vi "PH_AWG-510.Unpack Output Settings.vi"(2 "Output Settings":T1={"Activate Channel"=FALSE, "VPP (V)"=0.0, "Clock (Hz)"=0.0, "File Name (Device)"="", "#1"=0, "#2"=0, "#3"=0, "#4"=0, "#5"=0, "#6"=0, "#7"=0, "#8"=0, "#9"=0, "#10"=0, "#11"=0, "#12"=0, "#13"=0, "#14"=0, "#15"=0, "#16"=0, "#17"=0, "#18"=0, "#19"=0, "#20"=0, "Offset (V)"=-1.0} {"#20" max=1023 step=1 scale=0.0..1023.0; "#19" max=1023 step=1 scale=0.0..1023.0; "#18" max=1023 step=1 scale=0.0..1023.0; "#17" max=1023 step=1 scale=0.0..1023.0; "#16" max=1023 step=1 scale=0.0..1023.0; "#15" max=1023 step=1 scale=0.0..1023.0; "#14" max=1023 step=1 scale=0.0..1023.0; "#13" max=1023 step=1 scale=0.0..1023.0; "#12" max=1023 step=1 scale=0.0..1023.0; "#11" max=1023 step=1 scale=0.0..1023.0; "#10" max=1023 step=1 scale=0.0..1023.0; "#9" max=1023 step=1 scale=0.0..1023.0; "#8" max=1023 step=1 scale=0.0..1023.0; "#7" max=1023 step=1 scale=0.0..1023.0; "#6" max=1023 step=1 scale=0.0..1023.0; "#5" max=1023 step=1 scale=0.0..1023.0; "#4" max=1023 step=1 scale=0.0..1023.0; "#3" max=1023 step=1 scale=0.0..1023.0; "#2" max=1023 step=1 scale=0.0..1023.0; "#1" max=1023 step=1 scale=0.0..1023.0}) -> (14 "Activate Channel":bool, 15 "VPP [V]":dbl, 17 "Clock [Hz]":dbl, 18 "File Name (Device)":string, 19 "Waveform Pattern":u16[](array[numeric]))   [LabVIEW 2014, in "PH_AWG-510.lvlib"]
uses:
  PH_AWG-510.lvlib
  PH_AWG-510.Output Settings.ctl
panel:
  # "Waveform Pattern"
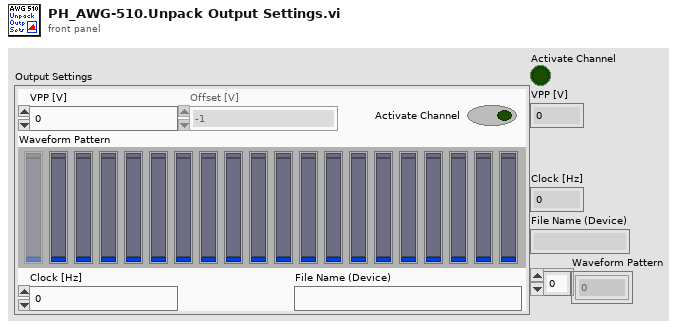
[diagram p1: front panel]
types:
  T1 = typedef "PH_AWG-510.lvlib/PH_AWG-510.Output Settings.ctl" = cluster{"Activate Channel":bool, "VPP (V)":dbl, "Clock (Hz)":dbl, "File Name (Device)":string, "#1":u16, "#2":u16, "#3":u16, "#4":u16, "#5":u16, "#6":u16, "#7":u16, "#8":u16, "#9":u16, "#10":u16, "#11":u16, "#12":u16, "#13":u16, "#14":u16, "#15":u16, "#16":u16, "#17":u16, "#18":u16, "#19":u16, "#20":u16, "Offset (V)":dbl}
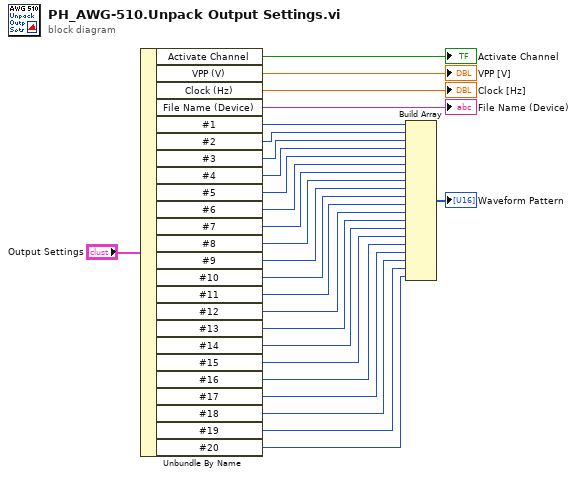
[diagram p0: block diagram]
diagram:
  n1 = Unbundle By Name("Output Settings") -> ("Activate Channel"=→"Activate Channel":bool, "VPP (V)"=→"VPP [V]":dbl, "Clock (Hz)"=→"Clock [Hz]":dbl, "File Name (Device)"=→"File Name (Device)":string, "#1"=w21:u16, "#2"=w20:u16, "#3"=w19:u16, "#4"=w18:u16, "#5"=w17:u16, "#6"=w16:u16, "#7"=w15:u16, "#8"=w14:u16, "#9"=w13:u16, "#10"=w12:u16, "#11"=w11:u16, "#12"=w10:u16, "#13"=w9:u16, "#14"=w8:u16, "#15"=w7:u16, "#16"=w6:u16, "#17"=w5:u16, "#18"=w4:u16, "#19"=w3:u16, "#20"=w2:u16)
  n2 = Build Array(w21, w20, w19, w18, w17, w16, w15, w14, w13, w12, w11, w10, w9, w8, w7, w6, w5, w4, w3, w2) -> (→"Waveform Pattern":u16[])
